vi "convert cell to dbl.vi"(8 "error in":errorcluster, 10 "start index":i32=6, 11 "Array":string[](array[string])) -> (0 "error out":errorcluster, 3 "Numeric of start index":dbl)   [LabVIEW 2016]
panel:
  out "size(s)":i32
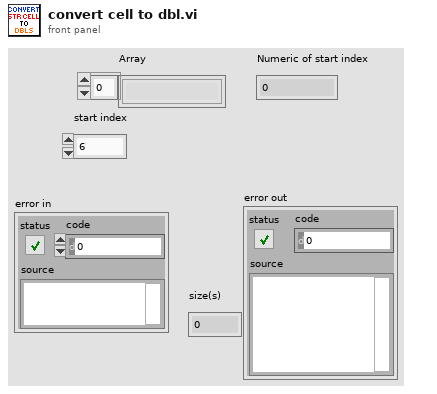
[diagram p1: front panel]
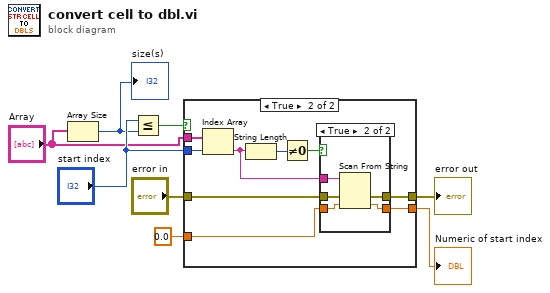
[diagram p0: block diagram]
diagram:
  n1 = Array Size(array="Array") -> (size(s)=w4:i32)
  "size(s)" <- w4
  n2 = Less Or Equal?(x="start index", y=w4) -> (x <= y?=w6:bool)
  n3 = case shown="True" w6 {
    tunnel: "start index" -> [_ w19]
    tunnel: [w9 w18] -> w8
    tunnel: "error in" -> [w10 w17]
    tunnel: 0.0 ("default value 1") -> [w9 w16]
    tunnel: [w10 w15] -> w1
    tunnel: "Array" -> [_ w14]
    frame False {
    }
    frame True {
      n4 = Index Array(array=w14, index=w19) -> (element=w13:string)
      n5 = String Length(string=w13) -> (length=w12:i32)
      n6 = Not Equal To 0?(x=w12) -> (x != 0?=w11:bool)
      n7 = case shown="True" w11 {
        tunnel: w13 -> [_ w26]
        tunnel: [w20 w25] -> w18
        tunnel: w17 -> [w21 w24]
        tunnel: w16 -> [w20 w23]
        tunnel: [w21 w22] -> w15
        frame False {
        }
        frame True {
          n8 = Scan From String(input string=w26, error in=w24, default 1=w23) -> (error out=w22:errorcluster, output 1=w25:dbl)  [unwired: 2 in, 2 out]
        }
      }
    }
  }
  "Numeric of start index" <- w8
  "error out" <- w1
